vi "WPI_UltrasonicRefNum Registry Set.vi"   [LabVIEW 2017]
doc: "Sets a reference into a registry so that other VIs can call the reference. After you set a reference, you can call that reference with the RefNum Registry Get VI."
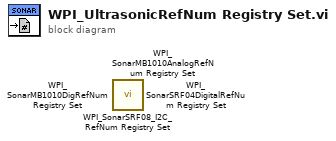
[diagram p0: block diagram]
diagram:
  n1 = call <vilib>:"WPI_SonarSRF08_I2C_RefNum Registry Set.vi"() -> ()  [unwired: 10 in, 2 out]
  n2 = call <vilib>:"WPI_SonarMB1010AnalogRefNum Registry Set.vi"() -> ()  [unwired: 10 in, 2 out]
  n3 = call <vilib>:"WPI_SonarMB1010DigRefNum Registry Set.vi"() -> ()  [unwired: 10 in, 2 out]
  n4 = call <vilib>:"WPI_SonarSRF04DigitalRefNum Registry Set.vi"() -> ()  [unwired: 10 in, 2 out]
